vi "SetComparisonType.vi"(8 "error in":errorcluster, 10 "ComparisonType":T1, 11 "IntegerMeasureLimit in":refnum<class "IntegerMeasureLimit.lvclass">) -> (0 "error out":errorcluster, 3 "IntegerMeasureLimit out":refnum<class "IntegerMeasureLimit.lvclass">)   [LabVIEW 2021, in "ProligentXMLGenerator.lvlib" / "IntegerMeasureLimit.lvclass"]
doc: "Real Measure Limit Comparison Type"
uses:
  IntegerMeasureLimit.lvclass
  IntegerMeasureLimit.lvclass/IntegerMeasureLimit.ctl
  Base/Integer/Integer.lvclass
  RangeMeasureLimit/RangeMeasureLimit.lvclass
  RangeMeasureLimit/ComparisonType.ctl
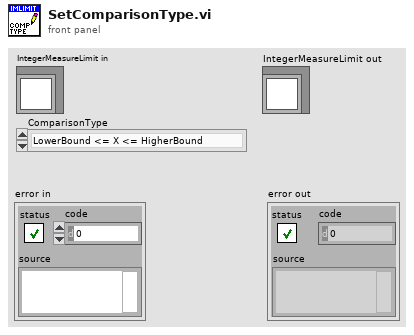
[diagram p1: front panel]
types:
  T1 = typedef "ProligentXMLGenerator.lvlib/RangeMeasureLimit.lvclass/ComparisonType.ctl" = enum16{"LowerBound <= X <= HigherBound", "LowerBound < X <= HigherBound", "LowerBound <= X < HigherBound", "LowerBound < X < HigherBound", "LowerBound <= X", "LowerBound < X", "X <= HigherBound", "X < HigherBound", "X == HigherBound", "X != HigherBound", "X <= LowerBound OR HigherBound <= X", "X < LowerBound OR HigherBound <= X", "X <= LowerBound OR HigherBound < X", "X < LowerBound OR HigherBound < X"}
  T2 = typedef "ProligentXMLGenerator.lvlib/IntegerMeasureLimit.lvclass/Data.ctl" = cluster{"LowerBound":refnum<class "Integer.lvclass">, "HigherBound":refnum<class "Integer.lvclass">}
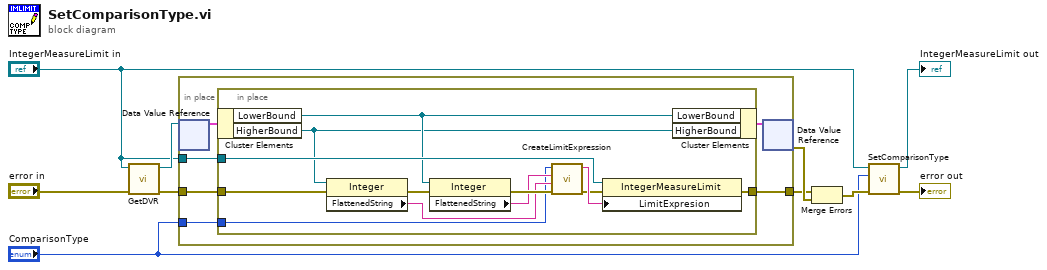
[diagram p0: block diagram]
diagram:
  n1 = call "GetDVR.vi"("error in"="error in", "IntegerMeasureLimit"="IntegerMeasureLimit in") -> ("error out"=w8:errorcluster, "DVRReference"=w9:refnum<data-value>)  [unwired: 8 in]
  n2 = in-place "In Place Element Structure" {
    in-place-border: "ComparisonType" -> [w16]
    in-place-border: w8 -> [w13]
    in-place-border: [w12] -> w6
    in-place-border: "IntegerMeasureLimit in" -> [w11]
    n3 = in-place-dvr #1(w9) -> (w15:T2)  [unwired: 1 out]
    n4 = in-place "In Place Element Structure" {
      in-place-border: w16 -> [w17]
      in-place-border: w13 -> [w28]
      in-place-border: [w24] -> w12
      in-place-border: w11 -> [w27]
      n5 = in-place-cluster #2(w15) -> ("LowerBound"=w19:refnum<class "Integer.lvclass">, "HigherBound"=w18:refnum<class "Integer.lvclass">)
      n6 = property class="Integer"(reference=w18, error in=w28) -> (error out=w23:errorcluster, "FlattenedString"=w21:string)  [unwired: 1 out]
      n7 = property class="Integer"(reference=w19, error in=w23) -> (error out=w22:errorcluster, "FlattenedString"=w20:string)  [unwired: 1 out]
      n8 = call "CreateLimitExpression.vi"("error in"=w22, "HigherBound"=w21, "LowerBound"=w20, "ComparisonType"=w17) -> ("error out"=w25:errorcluster, "LimitExpression"=w26:string)  [unwired: 6 in]
      n9 = property class="IntegerMeasureLimit"(reference=w27, error in=w25, "LimitExpresion"=w26) -> (error out=w24:errorcluster)  [unwired: 1 out]
      n10 = in-place-cluster #2("LowerBound"=w19, "HigherBound"=w18) -> (w14:T2)
    }
    n11 = in-place-dvr #1(w14) -> (w7:errorcluster)  [unwired: 1 out]
  }
  n12 = Merge Errors(w6, w7) -> (w5:errorcluster)
  n13 = call-parent "SetComparisonType.vi"("error in"=w5, "ComparisonType"="ComparisonType", "RangeMeasureLimit in"="IntegerMeasureLimit in") -> ("error out"=→"error out":errorcluster, "RangeMeasureLimit out"=→"IntegerMeasureLimit out":refnum<class "IntegerMeasureLimit.lvclass">)  [unwired: 7 in]
